vi "Initialize RFFE.vi"(8 "error in (no error)":errorcluster, 10 "write buffer":string="5", 11 "Select Com Port":refnum<visa-resource-name>="COM1") -> (0 "error out":errorcluster, 3 "VISA resource name out":refnum<visa-resource-name>)   [LabVIEW 2017]
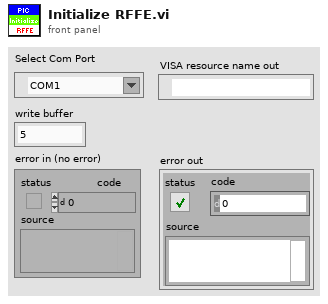
[diagram p1: front panel]
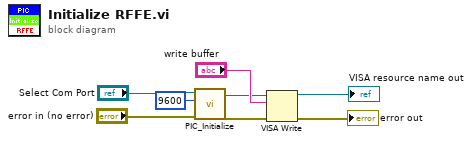
[diagram p0: block diagram]
diagram:
  n1 = call "PIC_Initialize.vi"("error in (no error)"="error in (no error)", "baud rate"=u32 9600, "Select Com Port"="Select Com Port") -> ("error out"=w7:errorcluster, "VISA resource name out"=w6:refnum<visa-resource-name>)  [unwired: 7 in]
  n2 = VISA Write(VISA resource name=w6, write buffer="write buffer", error in (no error)=w7) -> (VISA resource name out=→"VISA resource name out":refnum<visa-resource-name>, error out=→"error out":errorcluster)  [unwired: 1 out]
